vi "Initialize Device.vi"(7 "Baud Rate Override":u32, 8 "Error In":errorcluster, 9 "TCP Configuration":T3, 10 "COM Port":refnum<visa-resource-name>, 11 "Interface":T2) -> (0 "Error Out":errorcluster, 3 "LINX Device Config":T1)   [LabVIEW 2014, in "LMH-LINX.lvlib" / "Device.lvlib"]
doc: "Open a connection to the LINX device."
uses:
  Device.lvlib
  Type Defs/TCP Config.ctl
  Type Defs/Interface.ctl
  Type Defs/LINX Device Config.ctl
  Type Defs/Channels.ctl
  Type Defs/Packet Number FGV Action.ctl
  LMH-LINX.lvlib
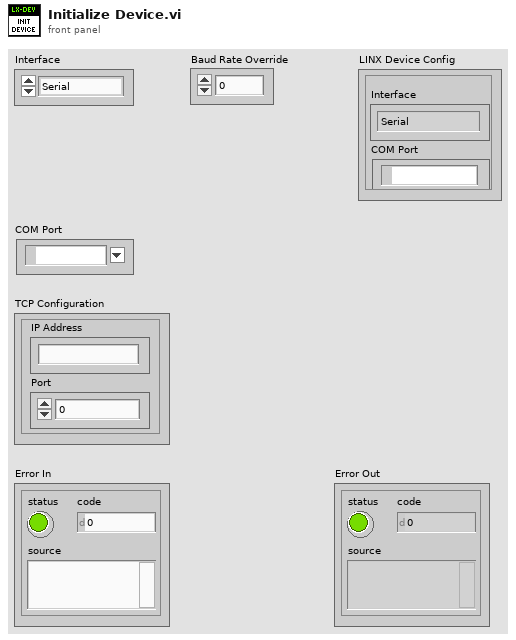
[diagram p1: front panel]
types:
  T1 = typedef "LMH-LINX.lvlib/Device.lvlib/LINX Device Config.ctl" = cluster{"Interface":T2, "COM Port":refnum<visa-resource-name>, "TCP Configuration":T3, "Device Family":u8, "Device ID":u8, "Device Name":string, "TCP Ref":refnum<k5>, "Channels":T4}
  T2 = typedef "LMH-LINX.lvlib/Interface.ctl" = enum16{"Serial", "TCP"}
  T3 = typedef "LMH-LINX.lvlib/Device.lvlib/TCP Config.ctl" = cluster{"IP Address":string, "Port":u16}
  T4 = typedef "LMH-LINX.lvlib/Channels.ctl" = cluster{"DI":u8[], "DO":u8[], "AI":u8[], "AO":u8[], "PWM":u8[], "QE":u8[], "UART":u8[], "I2C 2":u8[], "SPI":u8[], "CAN":u8[], "Servo":u8[], "AI Ref (V)":dbl, "AO Ref (V)":dbl, "AO Resolution (Bits)":u8}
  T5 = typedef "LMH-LINX.lvlib/Device.lvlib/Packet Number FGV Action.ctl" = enum16{"Initialize", "Get", "Increment"}
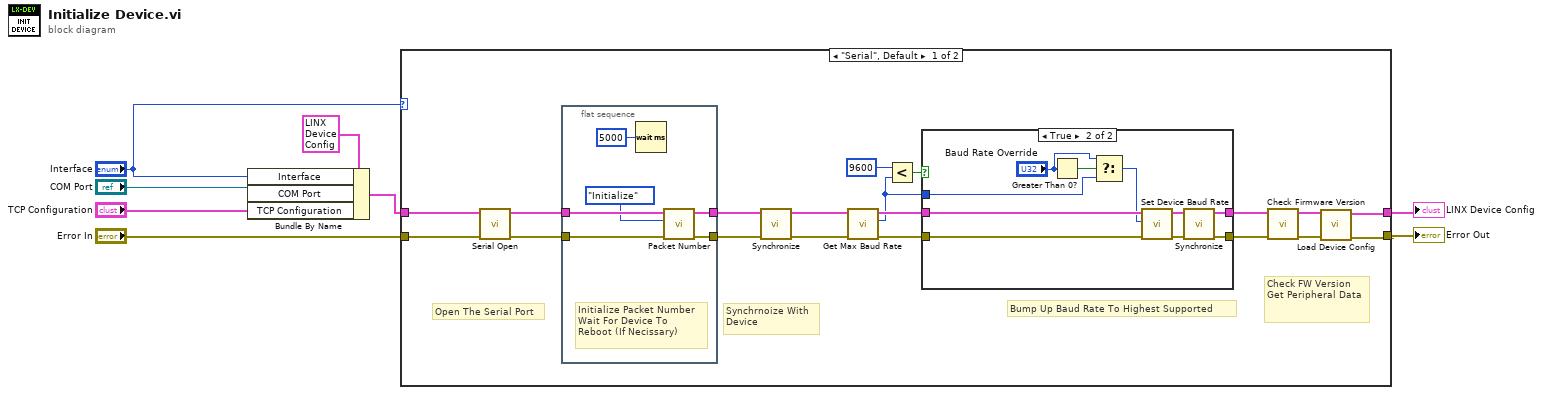
[diagram p0: block diagram]
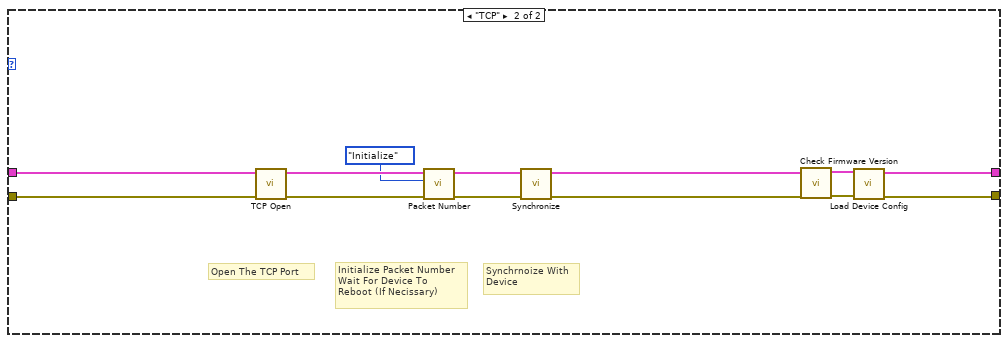
[diagram p3: hidden frame]
diagram:
  n1 = Bundle By Name(cluster=T1 {"Interface"=enum."Serial", "COM Port"="", "TCP Configuration"={"IP Address"="", "Port"=0}, "Device Family"=0, "Device ID"=0, "Device Name"="", "TCP Ref"=refnum, "Channels"={"DI"=[], "DO"=[], "AI"=[], "AO"=[], "PWM"=[], "QE"=[], "UART"=[], "I2C 2"=[], "SPI"=[], "CAN"=[], "Servo"=[], "AI Ref (V)"=0.0, "AO Ref (V)"=0.0, "AO Resolution (Bits)"=0}} ("LINX Device Config"), "Interface"="Interface", "COM Port"="COM Port", "TCP Configuration"="TCP Configuration") -> (w3:T1)
  n2 = case shown="\"Serial\", Default" "Interface" {
    tunnel: "Error In" -> [w27 w58]
    tunnel: [w20 w51] -> w1
    tunnel: w3 -> [w26 w57]
    tunnel: [w21 w52] -> w2
    frame "Serial", Default {
      # "Check FW Version\nGet Peripheral Data"
      # "Bump Up Baud Rate To Highest Supported"
      # "Synchrnoize With\nDevice"
      # "Open The Serial Port"
      n3 = call "Serial Open.vi"("Error In"=w27, "LINX Device Config"=w26) -> ("Error Out"=w22:errorcluster, "LINX Device Config"=w25:T1)  [unwired: 8 in]
      n4 = flat-sequence {
        tunnel: w25 -> [w33]
        tunnel: [w32] -> w24
        tunnel: [w31] -> w23
        tunnel: w22 -> [w30]
        frame #0 {
          # "Initialize Packet Number\nWait For Device To \nReboot (If Necissary)"
          n5 = Wait (ms)(milliseconds to wait=u32 5000) -> ()  [unwired: 1 out]
          n6 = call "Packet Number.vi"("Error In"=w30, "Action"=Packet_Number_FGV_Action."Initialize", "LINX Device Config"=w33) -> ("Error Out"=w31:errorcluster, "LINX Device Config"=w32:T1)  [unwired: 6 in, 1 out]
        }
      }
      n7 = call "Synchronize.vi"("Error In"=w23, "LINX Device Config"=w24) -> ("Error Out"=w18:errorcluster, "LINX Device Config"=w19:T1)  [unwired: 8 in]
      n8 = call "Get Max Baud Rate.vi"("Error In"=w18, "LINX Device Config"=w19) -> ("Error Out"=w14:errorcluster, "Baud Rate"=w11:u32, "LINX Device Config"=w15:T1)  [unwired: 7 in]
      n9 = Less?(x=u32 9600 ("y"), y=w11) -> (x < y?=w12:bool)
      n10 = case shown="True" w12 {
        tunnel: w15 -> [w35 w45]
        tunnel: w14 -> [w34 w44]
        tunnel: [w35 w41] -> w17
        tunnel: [w34 w40] -> w16
        tunnel: w11 -> [_ w37]
        frame False {
          # "No Faster Baud Rates Supported"
        }
        frame True {
          n11 = Greater Than 0?(x="Baud Rate Override") -> (x > 0?=w38:bool)
          n12 = Select(t="Baud Rate Override", s=w38, f=w37) -> (s? t:f=w36:u32)
          n13 = call "Set Device Baud Rate.vi"("Error In"=w44, "Baud Rate"=w36, "LINX Device Config"=w45) -> ("Error Out"=w42:errorcluster, "LINX Device Config"=w43:T1)  [unwired: 6 in, 1 out]
          n14 = call "Synchronize.vi"("Error In"=w42, "LINX Device Config"=w43) -> ("Error Out"=w40:errorcluster, "LINX Device Config"=w41:T1)  [unwired: 8 in]
        }
      }
      n15 = call "Check Firmware Version.vi"("Error In"=w16, "LINX Device Config"=w17) -> ("Error Out"=w10:errorcluster, "LINX Device Config"=w9:T1)  [unwired: 8 in]
      n16 = call "Load Device Config.vi"("Error In"=w10, "LINX Device Config"=w9) -> ("Error Out"=w20:errorcluster, "LINX Device Config"=w21:T1)  [unwired: 8 in]
    }
    frame "TCP" {
      # "Synchrnoize With\nDevice"
      # "Initialize Packet Number\nWait For Device To \nReboot (If Necissary)"
      # "Open The TCP Port"
      n17 = call "TCP Open.vi"("Error In"=w58, "LINX Device Config"=w57) -> ("Error Out"=w53:errorcluster, "LINX Device Config"=w56:T1)  [unwired: 8 in]
      n18 = call "Packet Number.vi"("Error In"=w53, "Action"=Packet_Number_FGV_Action."Initialize", "LINX Device Config"=w56) -> ("Error Out"=w54:errorcluster, "LINX Device Config"=w55:T1)  [unwired: 6 in, 1 out]
      n19 = call "Synchronize.vi"("Error In"=w54, "LINX Device Config"=w55) -> ("Error Out"=w46:errorcluster, "LINX Device Config"=w47:T1)  [unwired: 8 in]
      n20 = call "Check Firmware Version.vi"("Error In"=w46, "LINX Device Config"=w47) -> ("Error Out"=w49:errorcluster, "LINX Device Config"=w48:T1)  [unwired: 8 in]
      n21 = call "Load Device Config.vi"("Error In"=w49, "LINX Device Config"=w48) -> ("Error Out"=w51:errorcluster, "LINX Device Config"=w52:T1)  [unwired: 8 in]
    }
  }
  "Error Out" <- w1
  "LINX Device Config" <- w2
